vi "Extract.vi"(8 "error in (no error)":errorcluster, 11 "VisionUI in":refnum<class "VisionUI.lvclass">) -> (0 "error out":errorcluster, 3 "VisionUI out":refnum<class "VisionUI.lvclass">)   [LabVIEW 2019, in "VisionUI.lvlib" / "VisionUI.lvclass"]
uses:
  VisionUI.lvclass
  C:/Repos/Demo/Actors/Vision/Vision/Vision.lvclass
  VisionUI.lvclass/VisionUI.ctl
  Vision/Vision/Vision.lvclass
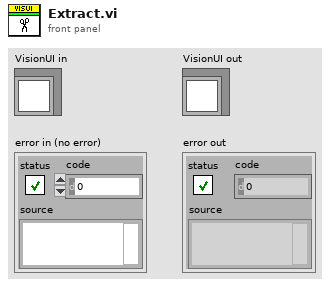
[diagram p1: front panel]
types:
  T1 = typedef "IMAQ Image.ctl" = refnum<image>
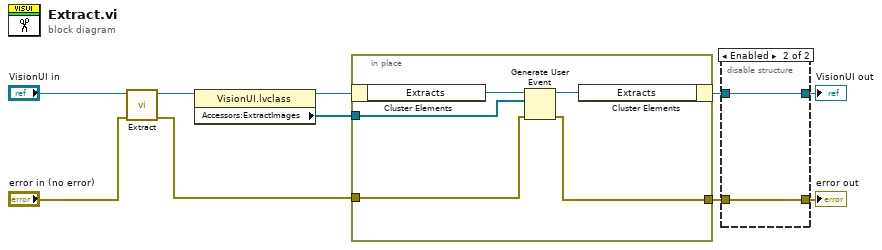
[diagram p0: block diagram]
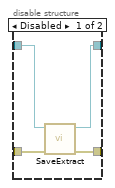
[diagram p2: hidden frame]
diagram:
  n1 = call-parent "Extract.vi"("error in (no error)"="error in (no error)", "Vision in"="VisionUI in") -> ("error out"=w6:errorcluster, "Vision out"=w10:refnum<class "VisionUI.lvclass">)  [unwired: 8 in]
  n2 = property class="VisionUI.lvclass"(reference=w10) -> (reference out=w7:refnum<class "VisionUI.lvclass">, "Accessors:ExtractImages"=w5:T1[])  [unwired: 1 in, 1 out]
  n3 = in-place {
    in-place-border: w6 -> [w13]
    in-place-border: [w12] -> w3
    in-place-border: w5 -> [w11]
    n4 = in-place-cluster #1(w7) -> ("Extracts"=w15:refnum<user-event>)
    n5 = Generate User Event(user event=w15, event data cluster=w11, error in=w13) -> (user event out=w14:refnum<user-event>, error out=w12:errorcluster)  [unwired: 1 in]
    n6 = in-place-cluster #1("Extracts"=w14) -> (w4:refnum<class "VisionUI.lvclass">)
  }
  n7 = disable-structure shown="Enabled" {
    disable-tunnel: w4 -> [w19 w21]
    disable-tunnel: w3 -> [w18 w20]
    disable-tunnel: [w17 w21] -> w2
    disable-tunnel: [w16 w20] -> w1
    frame Disabled {
      n8 = call "SaveExtract.vi"("error in (no error)"=w18, "VisionUI in"=w19) -> ("error out"=w16:errorcluster, "VisionUI out"=w17:refnum<class "VisionUI.lvclass">)  [unwired: 8 in]
    }
    frame Enabled {
    }
  }
  "error out" <- w1
  "VisionUI out" <- w2
